vi "Run - Array of Status Monitors With Transient Captures.vi"() -> ()   [LabVIEW 2017]
panel:
  in  "List of INI Files":path[](array[path])
  in  "Pre-Trigger Samples":i32
  in  "Post-Trigger Samples":i32
  in  "Soft Trigger":bool
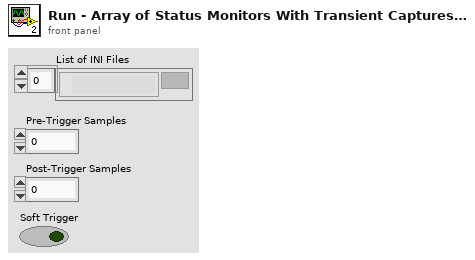
[diagram p1: front panel]
types:
  T1 = enum32{"Invalid", "Standard", "Closed", "Hidden", "Minimized", "Maximized"}
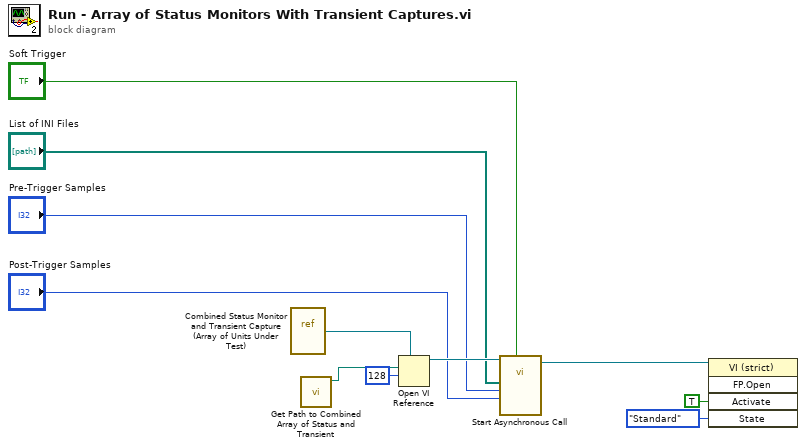
[diagram p0: block diagram]
diagram:
  n1 = vi-ref "Combined Status Monitor and Transient Capture (Array of Units Under Test).vi"() -> (w11:refnum<vi>)
  n2 = call "Get Path to Combined Array of Status and Transient.vi"() -> ("Path to Combined Status and Transient"=w10:path)  [unwired: 11 in]
  n3 = Open VI Reference(type specifier VI Refnum (for type only)=w11, vi path=w10, options=128) -> (vi reference=w8:refnum<vi>)  [unwired: 3 in, 1 out]
  n4 = call-by-ref "Start Asynchronous Call"(reference=w8, "Soft Trigger"="Soft Trigger", "Post-Trigger Samples"="Post-Trigger Samples", "Pre-Trigger Samples"="Pre-Trigger Samples", "List of INI Files"="List of INI Files") -> (reference out=w3:refnum<vi>)  [unwired: 9 in, 1 out]
  n5 = invoke class="VI (strict)" method="FP.Open"(reference=w3, "Activate"=TRUE ("Activate?"), "State"=T1."Standard") -> ()  [unwired: 2 in, 5 out]
